vi "ziImpedanceCalibApply.vi"(4 "Calib Phase (T)":bool=TRUE, 5 "Calib Amplitude (T)":bool=TRUE, 7 "Measurement":cdb[](array[numeric]), 8 "Frequencies (Hz)":dbl[](array[numeric]), 9 "ziCalib In":T1) -> (1 "Corrected Measurement":cdb[](array[numeric]), 2 "Extrapolated":bool, 3 "ziCalib Out":T1)   [LabVIEW 2009, in "Zurich Instruments LabOne.lvlib"]
doc: "Apply a calibration obtained with ziImpedanceCalibObtain.vi to a measurement."
uses:
  <instrlib>/Zurich Instruments LabOne/Zurich Instruments LabOne.lvlib
  <instrlib>/Zurich Instruments LabOne/Public/Utility/Impedance/ziTypeCalib.ctl
  <instrlib>/Zurich Instruments LabOne/Public/Utility/Impedance/ziTypeCalibModel.ctl
  <instrlib>/Zurich Instruments LabOne/Public/Utility/Impedance/ziTypeImpedanceEqCircModel.ctl
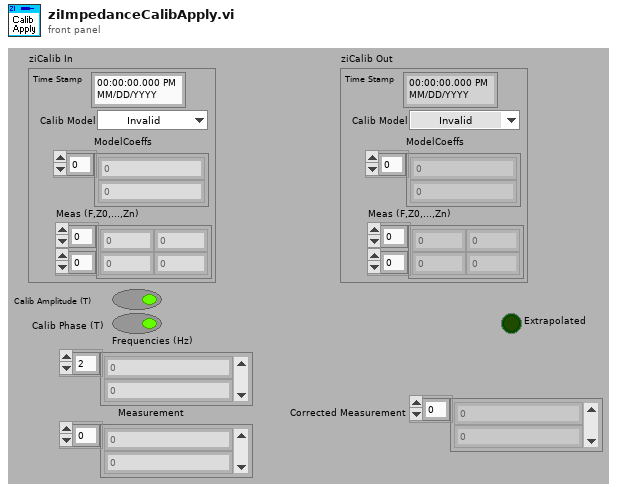
[diagram p1: front panel]
types:
  T1 = typedef "Zurich Instruments LabOne.lvlib/ziTypeCalib.ctl" = cluster{"Time Stamp":timestamp, "Calib Model":T2, "ModelCoeffs":cdb[], "Meas (F,Z0,...,Zn)":dbl[][]}
  T2 = typedef "Zurich Instruments LabOne.lvlib/ziTypeCalibModel.ctl" = enum16{"Invalid", "Unity", "R||C", "R||L", "R*C", "R*L"}
  T3 = typedef "Zurich Instruments LabOne.lvlib/ziTypeImpedanceEqCircModel.ctl" = enum16{"Invalid", "|Z|, Phi", "R||C", "R||L", "R*C", "D*C", "R*L", "ReZ, ImZ", "G, B"}
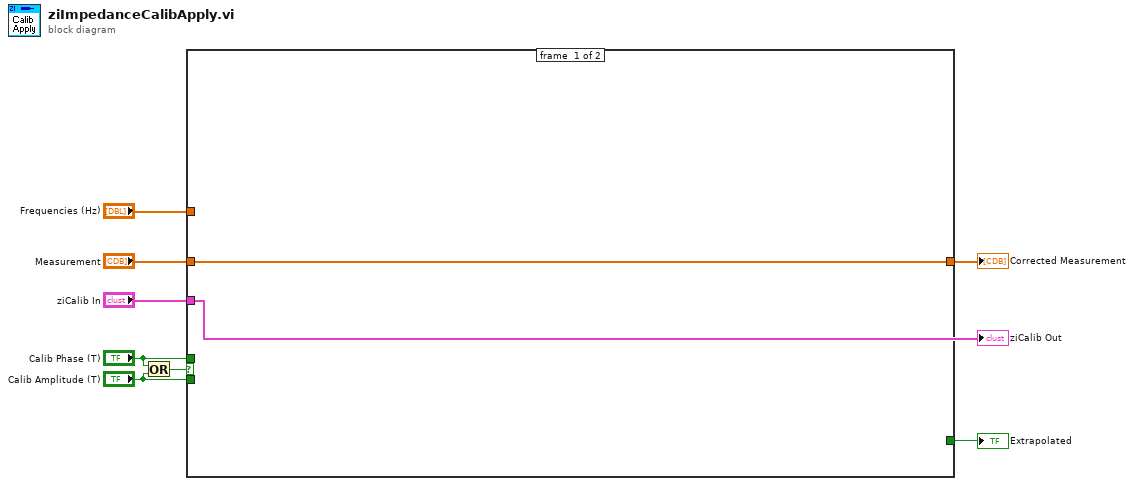
[diagram p0: block diagram]
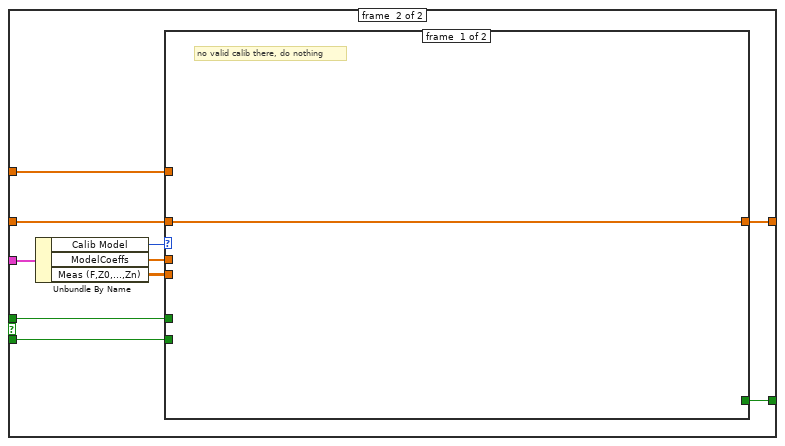
[diagram p2: hidden frame]
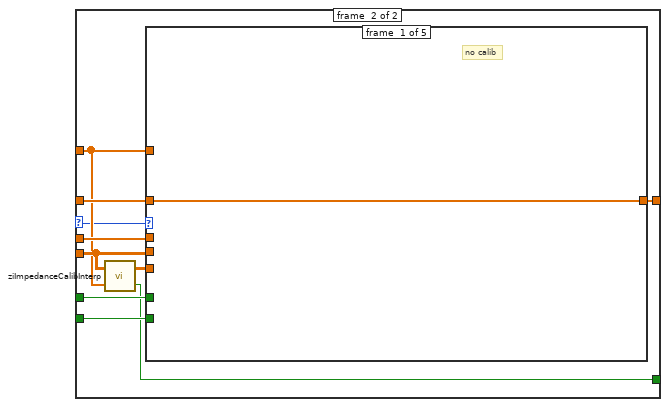
[diagram p3: hidden frame]
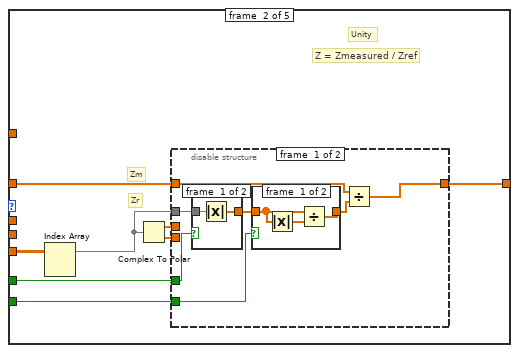
[diagram p4: hidden frame]
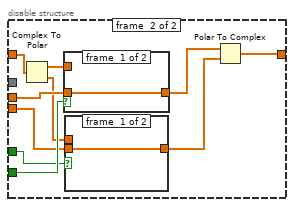
[diagram p7: hidden frame]
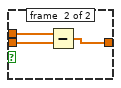
[diagram p8: hidden frame]
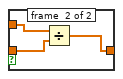
[diagram p9: hidden frame]
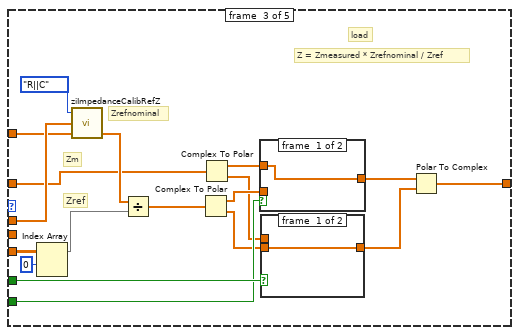
[diagram p10: hidden frame]
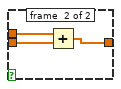
[diagram p11: hidden frame]
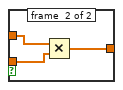
[diagram p12: hidden frame]
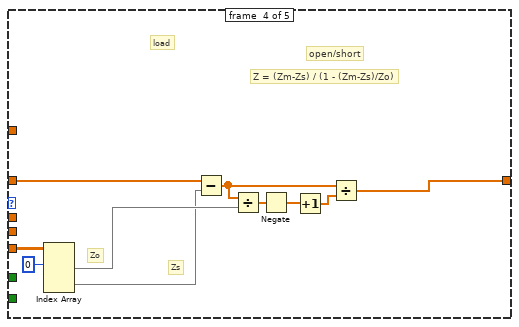
[diagram p13: hidden frame]
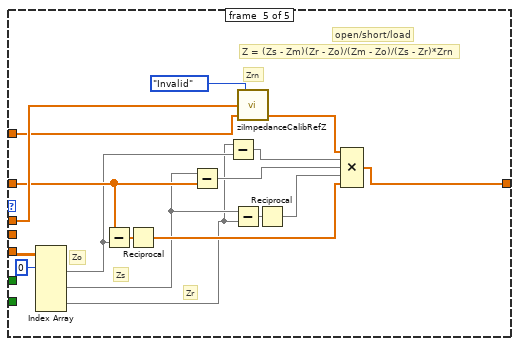
[diagram p14: hidden frame]
diagram:
  n1 = Or(x="Calib Phase (T)", y="Calib Amplitude (T)") -> (x .or. y?=w2:bool)
  n2 = case shown="True" w2 {
    tunnel: "Frequencies (Hz)" -> [_ w12]
    tunnel: "Measurement" -> [w9 w19]
    tunnel: [w9 w18] -> w6
    tunnel: "ziCalib In" -> [_ w16]
    tunnel: "Calib Phase (T)" -> [_ w15]
    tunnel: "Calib Amplitude (T)" -> [_ w14]
    tunnel: [_ w11] -> w1
    frame #0 {
    }
    frame #1 {
      n3 = Unbundle By Name(w16) -> ("Calib Model"=w10:T2, "ModelCoeffs"=w17:cdb[], "Meas (F,Z0,...,Zn)"=w13:dbl[][])
      n4 = case shown="Default" w10 {
        selector: w10 -> [_ w21]
        tunnel: w19 -> [w20 w30]
        tunnel: [w20 w29] -> w18
        tunnel: w17 -> [_ w28]
        tunnel: w15 -> [_ w27]
        tunnel: w14 -> [_ w26]
        tunnel: w13 -> [_ w25]
        tunnel: w12 -> [_ w24]
        tunnel: [_ w22] -> w11
        frame #0 {
          # "no valid calib there, do nothing"
        }
        frame #1 {
          n5 = call <instrlib>:"ziImpedanceCalibInterp.vi"("Frequencies (Hz)"=w24, "Measurement_Z (F,X0,Y0,...Xn,Yn)"=w25) -> ("Extrapolated"=w22:bool, "Interpolated_Z (Series,F)"=w23:cdb[][])
          n6 = case shown="\"R||C\"" w21 {
            tunnel: w28 -> [_ _ w89 _ w124]
            tunnel: w24 -> [_ _ w88 _ w123]
            tunnel: w25 -> [_ _ _ _ _]
            tunnel: w30 -> [w31 w39 w84 w107 w121]
            tunnel: [w31 w36 w85 w102 w108] -> w29
            tunnel: w27 -> [_ w38 w83 _ _]
            tunnel: w26 -> [_ w37 w82 _ _]
            tunnel: w23 -> [_ w33 w86 w101 w113]
            frame #0 {
              # "no calib"
            }
            frame #1 {
              # "Zm"
              # "Zr"
              # "Z = Zmeasured / Zref"
              # "Unity"
              n7 = Index Array(array=w33) -> (element=w32:cdb[])  [unwired: 2 in]
              n8 = Complex To Polar(r * e^(i*theta)=w32) -> (r=w35:dbl[], theta=w34:dbl[])
              n9 = disable-structure shown="Enabled" {
                disable-tunnel: w39 -> [w46 w57]
                disable-tunnel: w38 -> [w43 w60]
                disable-tunnel: w37 -> [w42 w61]
                disable-tunnel: [w41 w55] -> w36
                disable-tunnel: w32 -> [w40 _]
                disable-tunnel: w35 -> [_ w63]
                disable-tunnel: w34 -> [_ w59]
                frame #0 {
                  n10 = case shown="False" w43 {
                    tunnel: w40 -> [w52 w53]
                    tunnel: [w51 w53] -> w45
                    frame #0 {
                      n11 = Absolute Value(x=w52) -> (abs(x)=w51:dbl[])
                    }
                    frame #1 {
                    }
                  }
                  n12 = case shown="False" w42 {
                    tunnel: w45 -> [w49 w50]
                    tunnel: [w47 w50] -> w44
                    frame #0 {
                      n13 = Absolute Value(x=w49) -> (abs(x)=w48:dbl[])
                      n14 = Divide(x=w49, y=w48) -> (x/y=w47:cdb[])
                    }
                    frame #1 {
                    }
                  }
                  n15 = Divide(x=w46, y=w44) -> (x/y=w41:cdb[])
                }
                frame #1 {
                  n16 = Complex To Polar(r * e^(i*theta)=w57) -> (r=w56:dbl[], theta=w54:dbl[])
                  n17 = case shown="True" w61 {
                    tunnel: w63 -> [w68 w70]
                    tunnel: [w68 w69] -> w62
                    tunnel: w56 -> [_ w71]
                    frame #0 {
                    }
                    frame #1 {
                      n18 = Divide(x=w71, y=w70) -> (x/y=w69:dbl[])
                    }
                  }
                  n19 = case shown="True" w60 {
                    tunnel: w59 -> [w64 w66]
                    tunnel: [w64 w65] -> w58
                    tunnel: w54 -> [_ w67]
                    frame #0 {
                    }
                    frame #1 {
                      n20 = Subtract(x=w67, y=w66) -> (x-y=w65:dbl[])
                    }
                  }
                  n21 = Polar To Complex(1:w58, 2:w62) -> (0:w55:cdb[])
                }
              }
            }
            frame #2 {
              # "Zm"
              # "Zrefnominal"
              # "Zref"
              # "Z = Zmeasured * Zrefnominal / Zref"
              # "load"
              n22 = Index Array(array=w86, index (row)=0) -> (element=w73:cdb[])  [unwired: 1 in]
              n23 = call <instrlib>:"ziImpedanceCalibRefZ.vi"("Frequencies (Hz)"=w88, "Model Values"=w89, "Eq Model (Unity)"=ziTypeImpedanceEqCircModel."R||C" ("Eq Model ID (Unity)")) -> ("Z (Ohm)"=w87:cdb[])  [unwired: 1 in, 1 out]
              n24 = Divide(x=w87, y=w73) -> (x/y=w81:cdb[])
              n25 = Complex To Polar(r * e^(i*theta)=w81) -> (r=w80:dbl[], theta=w79:dbl[])
              n26 = Complex To Polar(r * e^(i*theta)=w84) -> (r=w76:dbl[], theta=w75:dbl[])
              n27 = case shown="True" w82 {
                tunnel: w80 -> [_ w96]
                tunnel: [w94 w95] -> w78
                tunnel: w76 -> [w94 w97]
                frame #0 {
                }
                frame #1 {
                  n28 = Multiply(x=w97, y=w96) -> (x*y=w95:dbl[])
                }
              }
              n29 = case shown="True" w83 {
                tunnel: w79 -> [w90 w92]
                tunnel: [w90 w91] -> w77
                tunnel: w75 -> [_ w93]
                frame #0 {
                }
                frame #1 {
                  n30 = Add(x=w93, y=w92) -> (x+y=w91:dbl[])
                }
              }
              n31 = Polar To Complex(1:w77, 2:w78) -> (0:w85:cdb[])
            }
            frame #3 {
              # "load"
              # "Z = (Zm-Zs) / (1 - (Zm-Zs)/Zo)"
              # "Zs"
              # "Zo"
              # "open/short"
              n32 = Index Array(array=w101, index (row) #1=0 ("index (row)")) -> (element #1=w99:cdb[], element #2=w98:cdb[])  [unwired: 3 in]
              n33 = Subtract(x=w107, y=w98) -> (x-y=w105:cdb[])
              n34 = Divide(x=w105, y=w99) -> (x/y=w106:cdb[])
              n35 = Negate(x=w106) -> (-x=w104:cdb[])
              n36 = Increment(x=w104) -> (x+1=w103:cdb[])
              n37 = Divide(x=w105, y=w103) -> (x/y=w102:cdb[])
            }
            frame #4 {
              # "Zr"
              # "Zs"
              # "Zo"
              # "Z = (Zs - Zm)(Zr - Zo)/(Zm - Zo)/(Zs - Zr)*Zrn"
              # "Zrn"
              # "open/short/load"
              n38 = Index Array(array=w113, index (row) #1=0 ("index (row)")) -> (element #1=w111:cdb[], element #2=w110:cdb[], element #3=w109:cdb[])  [unwired: 5 in]
              n39 = Subtract(x=w121, y=w111) -> (x-y=w122:cdb[])
              n40 = Reciprocal(x=w122) -> (1/x=w115:cdb[])
              n41 = Subtract(x=w110, y=w121) -> (x-y=w117:cdb[])
              n42 = Subtract(x=w109, y=w111) -> (x-y=w118:cdb[])
              n43 = Subtract(x=w110, y=w109) -> (x-y=w120:cdb[])
              n44 = call <instrlib>:"ziImpedanceCalibRefZ.vi"("Frequencies (Hz)"=w123, "Model Values"=w124, "Eq Model (Unity)"=ziTypeImpedanceEqCircModel."Invalid" ("Eq Model ID (Unity)")) -> ("Z (Ohm)"=w119:cdb[])  [unwired: 1 in, 1 out]
              n45 = Reciprocal(x=w120) -> (1/x=w116:cdb[])
              n46 = Compound Arithmetic op=MULTIPLY(w119, w118, w117, w116, w115) -> (w108:cdb[])
            }
          }
        }
      }
    }
  }
  "Corrected Measurement" <- w6
  "Extrapolated" <- w1
  "ziCalib Out" <- "ziCalib In"
